vi "LDA_classifier_Trainer_prior.vi"(5 "Matrix":T1, 6 "Non_target_Flash_order":i64[][](array[numeric]) caption="NonTarget_Flash_Order", 7 "Value":T1, 8 "Target_Flash_Order":i64[](array[numeric]), 9 "Brain_data_source":dbl[][](array[numeric]) caption="EEG_Raw_Data" format="%0.3f", 10 "samples per channel":i32=25, 11 "rate":dbl=500.0 caption="Rate" format="%0.2f") -> (0 "FP":dbl[](array[numeric]), 2 "TP":dbl[](array[numeric]))   [LabVIEW 2013]
uses:
  <vilib>/Analysis/Matrix/Datatypes/RealMatrix.ctl
  <vilib>/Analysis/3filter.llb/Filter Passband Type.ctl
  <vilib>/Analysis/baseanly.llb/Mean (DBL).vi
  <vilib>/Analysis/3filter.llb/Butterworth Filter (DBL).vi
  <vilib>/Analysis/Matrix/Numeric/Conversions/Array To Matrix - RA.vi
  <vilib>/Analysis/Matrix/Numeric/Multiply/Multiply - RM,RM.vi
  <vilib>/Analysis/Matrix/Numeric/Subtract/Subtract - RM,RM.vi
  <vilib>/Analysis/Matrix/Numeric/Conversions/Matrix To Array - RM.vi
  <vilib>/Analysis/NI_AALBase.lvlib
  <vilib>/Analysis/Matrix/NI_Matrix.lvlib
panel:
  out "Total Length 2":i32
  out "Total Length":i32
  out "#channel":i32
  out "LDA Parameters\nfor All channel all\nflash":dbl[][](array[numeric])
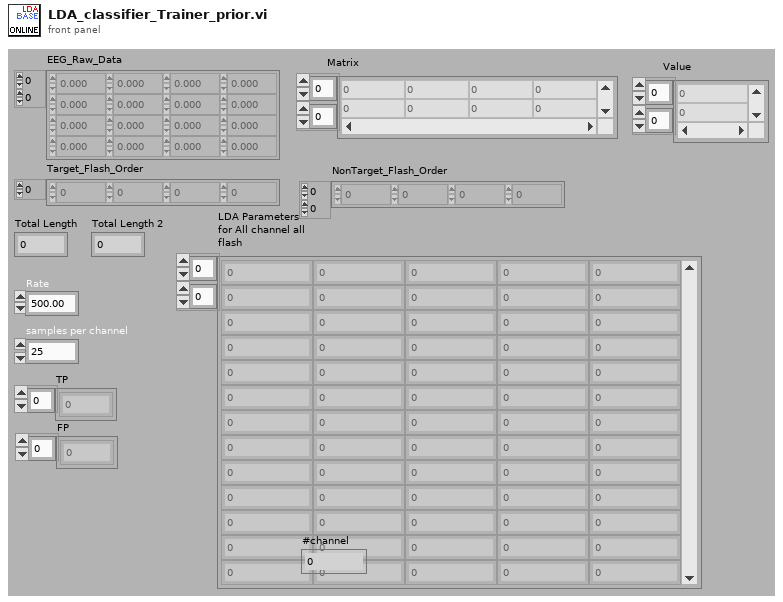
[diagram p1: front panel]
types:
  T1 = typedef "NI_Matrix.lvlib/RealMatrix.ctl" = dbl[][]
  T2 = typedef "NI_AALBase.lvlib/Filter Passband Type.ctl" = enum32{"Lowpass", "Highpass", "Bandpass", "Bandstop"}
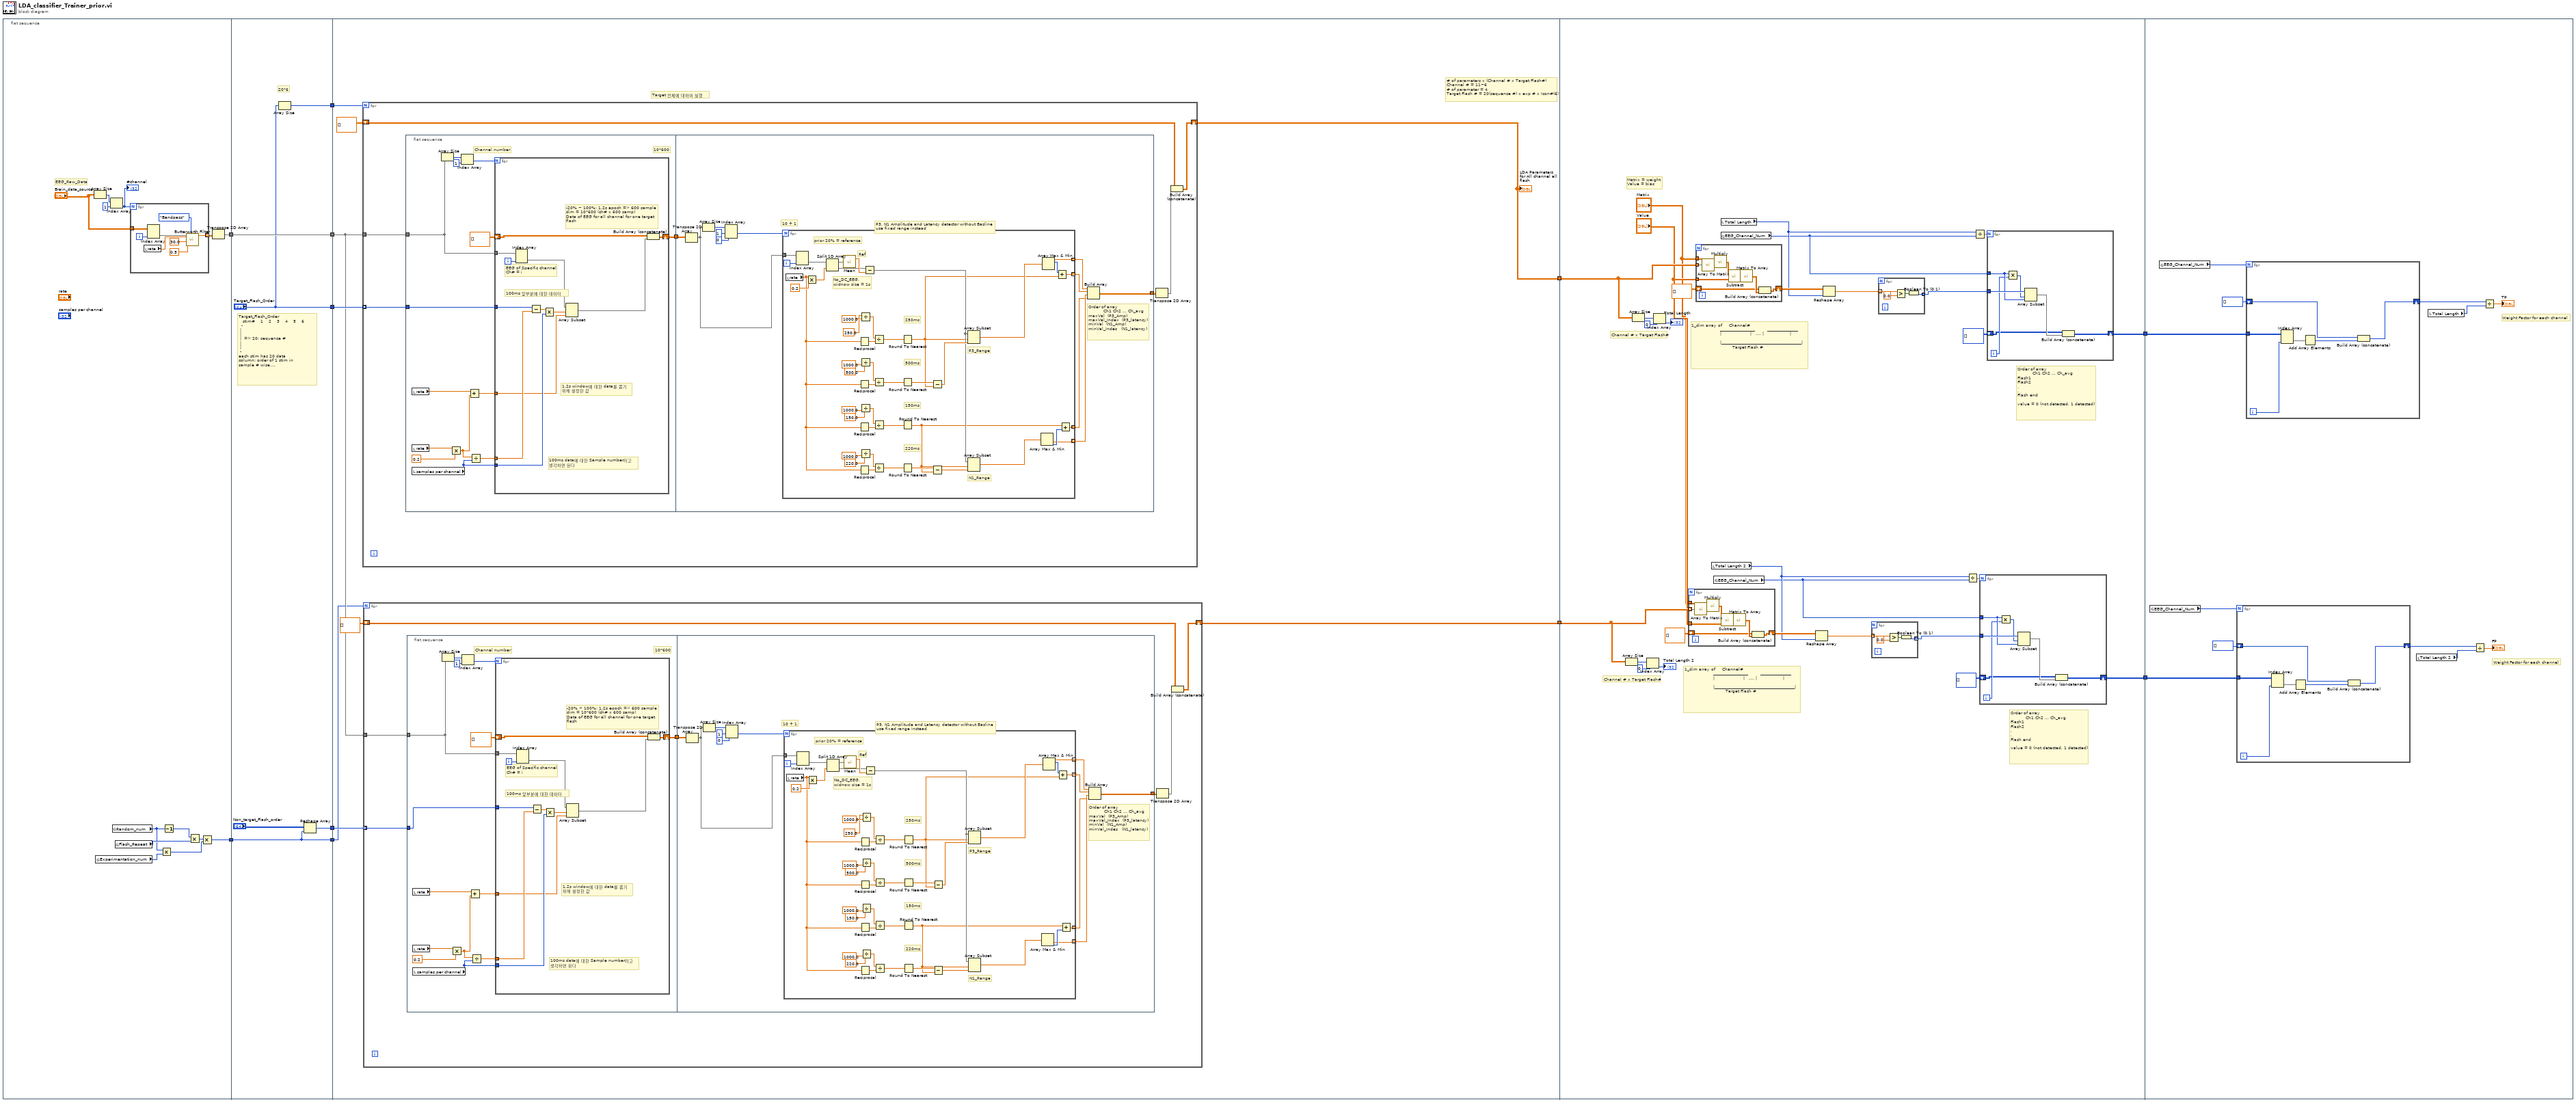
[diagram p0: block diagram]
diagram:
  n1 = flat-sequence {
    tunnel: [w20] -> w11
    tunnel: [w12] -> w2
    tunnel: [w38] -> w10
    tunnel: ["Target_Flash_Order"] -> w9
    tunnel: w11 -> [w38]
    tunnel: [w36] -> w7
    tunnel: [w34] -> w3
    tunnel: w2 -> [w33]
    tunnel: [w33] -> w1
    tunnel: w10 -> [w42]
    tunnel: w9 -> [w47]
    tunnel: [w45] -> w8
    tunnel: w7 -> [w44]
    tunnel: [w41] -> w5
    tunnel: w3 -> [w40]
    tunnel: w1 -> [w39]
    tunnel: w8 -> [w250]
    tunnel: [w239] -> w6
    tunnel: w5 -> [w227]
    tunnel: [w226] -> w4
    tunnel: w6 -> [w303]
    tunnel: w4 -> [w292]
    frame #0 {
      # "EEG_Raw_Data"
      n2 = Array Size(array="Brain_data_source") -> (size(s)=w21:i32[])
      n3 = global read "Control_Panel.vi" "Experimentation_num"() -> (w15:i32)
      n4 = Index Array(array=w21, index=1) -> (element=w23:i32)
      "#channel" <- w23
      n5 = global read "Control_Panel.vi" "Random_num"() -> (w16:i32)
      n6 = global read "Control_Panel.vi" "Flash_Repeat"() -> (w17:i32)
      n7 = for {
        N: w23 -> [_]
        tunnel: "Brain_data_source" -> [w32]
        tunnel: [w28] -> w24 mode=indexing
        i -> [w31]
        n8 = local read "rate"() -> (w25:dbl)
        n9 = Index Array(array=w32, index (col)=w31) -> (element=w30:dbl[])  [unwired: 1 in]
        n10 = call-poly <vilib>:"Butterworth Filter.vi"("filter type"=Filter_Passband_Type."Bandpass", "low cutoff freq: fl"=0.5, "high cutoff freq: fh"=30.0, "sampling freq: fs"=w25, "X"=w30) -> ("Filtered X"=w28:dbl[])  [unwired: 3 in, 1 out]
      }
      n11 = Multiply(x=w16, y=w15) -> (x*y=w13:i32)
      n12 = Decrement(x=w16) -> (x-1=w18:i32)
      n13 = Multiply(x=w18, y=w17) -> (x*y=w14:i32)
      n14 = Multiply(x=w14, y=w13) -> (x*y=w12:i32)
      n15 = Transpose 2D Array(2D array=w24) -> (transposed array=w20:dbl[][])
    }
    frame #1 {
      # "Target_Flash_Order\n   stim#    1    2    3    4    5    6    \n  -\n |\n |\n |  => 20: sequence # \n |\n |\n -\neach stim has 20 data\ncolumn: order of 1 stim in \nsample # wise...."
      # "20*6"
      n16 = Array Size(array="Target_Flash_Order") -> (size(s)=w36:i32)
      n17 = Reshape Array("Non_target_Flash_order", w33) -> (w34:i64[])
    }
    frame #2 {
      # "Target 전체에 대하여 실행"
      # "# of parameters x (Channel # x Target Flash#)\nChannel # = 11~6\n# of parameter = 4\nTarget Flash # = 20(sequence #) x exp # x Icon#(6)"
      n18 = for {
        N: w44 -> [_]
        tunnel: w42 -> [w141]
        tunnel: w47 -> [w136] mode=indexing
        shift-right: [w139] -> w45
        shift-left: dbl[][] [] -> [w138]
        n19 = flat-sequence {
          tunnel: w141 -> [w146]
          tunnel: [w145] -> w142
          tunnel: w136 -> [w144]
          tunnel: w142 -> [w172]
          tunnel: [w174] -> w137
          frame #0 {
            # "10*600"
            # "Channel number"
            n20 = local read "rate"() -> (w154:dbl)
            n21 = local read "rate"() -> (w152:dbl)
            n22 = local read "samples per channel"() -> (w143:i32)
            n23 = Array Size(array=w146) -> (size(s)=w148:i32[])
            n24 = Multiply(x=w152, y=0.2) -> (x*y=w156:dbl)
            n25 = Index Array(array=w148, index=1) -> (element=w150:i32)
            n26 = Add(x=w154, y=w156) -> (x+y=w155:dbl)
            n27 = Divide(x=w156, y=w143) -> (x/y=w153:dbl)
            n28 = for {
              N: w150 -> [_]
              tunnel: w155 -> [w158]
              shift-right: [w166] -> w145
              shift-left: dbl[][] [] -> [w167]
              tunnel: w146 -> [w165]
              tunnel: w153 -> [w162]
              tunnel: w144 -> [w163]
              tunnel: w143 -> [w159]
              i -> [w168]
              # "1.2s window에 대한 data를 뽑기\n위해 설정한 값"
              # "100ms data에 대한 Sample number라고 \n생각하면 된다"
              # "100ms 앞부분에 대한 데이터"
              # "EEG of Specific channel\nCh# = i"
              # "-20% ~ 100%: 1.2s epoch => 600 sample\ndim = 10*600 (ch# x 600 samp)\nData of EEG for all channel for one target \nflash"
              n29 = Index Array(array=w165, index (col)=w168) -> (element=w164:dbl[])  [unwired: 1 in]
              n30 = Subtract(x=w163, y=w162) -> (x-y=w161:dbl)
              n31 = Multiply(x=w161, y=w159) -> (x*y=w160:dbl)
              n32 = Array Subset(array=w164, index=w160, length=w158) -> (w157:dbl[])
              n33 = Build Array (concatenate)(w167, w157) -> (w166:dbl[][])
            }
          }
          frame #1 {
            # "P3, N1 Amplitude and Latency detector without Basline\nuse fixed range instead"
            # "Order of array\n           Ch1 Ch2 ... Ch_avg\nmaxVal  (P3_Amp)\nmaxVal_Index  (P3_latency)\nminVal  (N1_Amp)\nminVal_Indes   (N1_latency)"
            # "10 + 1"
            n34 = Transpose 2D Array(2D array=w172) -> (transposed array=w169:dbl[][])
            n35 = Array Size(array=w169) -> (size(s)=w173:i32[])
            n36 = Index Array(array=w173, index #1=1 ("index"), index #2=0 ("인덱스")) -> (element #1=w170:i32)  [unwired: 1 out]
            n37 = for {
              N: w170 -> [_]
              tunnel: w169 -> [w223]
              tunnel: [w218] -> w178 mode=indexing
              tunnel: [w216] -> w177 mode=indexing
              tunnel: [w213] -> w176 mode=indexing
              tunnel: [w212] -> w175 mode=indexing
              i -> [w211]
              # "N1_Range"
              # "P3_Range"
              # "220ms"
              # "150ms"
              # "500ms"
              # "250ms"
              # "No_DC_EEG,\nwidnow size = 1s"
              # "Ref"
              # "prior 20% = reference"
              n38 = local read "rate"() -> (w193:dbl)
              n39 = Index Array(array=w223, index (col)=w211) -> (element=w215:dbl[])  [unwired: 1 in]
              n40 = Multiply(x=w193, y=0.2) -> (x*y=w221:dbl)
              n41 = Split 1D Array(array=w215, index=w221) -> (first subarray=w220:dbl[], second subarray=w210:dbl[])
              n42 = call-poly <vilib>:"Mean.vi"("X"=w220) -> ("mean"=w219:dbl)  [unwired: 1 out]
              n43 = Reciprocal(x=w193) -> (1/x=w209:dbl)
              n44 = Reciprocal(x=w193) -> (1/x=w208:dbl)
              n45 = Reciprocal(x=w193) -> (1/x=w207:dbl)
              n46 = Reciprocal(x=w193) -> (1/x=w206:dbl)
              n47 = Divide(x=250.0, y=1000.0) -> (x/y=w205:dbl)
              n48 = Divide(x=500.0, y=1000.0) -> (x/y=w204:dbl)
              n49 = Divide(x=150.0, y=1000.0) -> (x/y=w203:dbl)
              n50 = Divide(x=220.0, y=1000.0) -> (x/y=w202:dbl)
              n51 = Subtract(x=w210, y=w219) -> (x-y=w184:dbl[])
              n52 = Divide(x=w205, y=w209) -> (x/y=w192:dbl)
              n53 = Divide(x=w204, y=w208) -> (x/y=w191:dbl)
              n54 = Divide(x=w203, y=w207) -> (x/y=w190:dbl)
              n55 = Divide(x=w202, y=w206) -> (x/y=w189:dbl)
              n56 = Round To Nearest(number=w192) -> (nearest integer value=w181:dbl)
              n57 = Round To Nearest(number=w191) -> (nearest integer value=w186:dbl)
              n58 = Round To Nearest(number=w190) -> (nearest integer value=w180:dbl)
              n59 = Round To Nearest(number=w189) -> (nearest integer value=w188:dbl)
              n60 = Subtract(x=w186, y=w181) -> (x-y=w185:dbl)
              n61 = Subtract(x=w188, y=w180) -> (x-y=w187:dbl)
              n62 = Array Subset(array=w184, index=w181, length=w185) -> (w182:dbl[])
              n63 = Array Subset(array=w184, index=w180, length=w187) -> (w183:dbl[])
              n64 = Array Max & Min(array=w183) -> (min value=w213:dbl, min index (indices)=w214:i32)  [unwired: 2 out]
              n65 = Array Max & Min(array=w182) -> (max value=w218:dbl, max index (indices)=w217:i32)  [unwired: 2 out]
              n66 = Add(x=w217, y=w181) -> (x+y=w216:dbl)
              n67 = Add(x=w180, y=w214) -> (x+y=w212:dbl)
            }
            n68 = Build Array(w178, w177, w176, w175) -> (w174:dbl[][])
          }
        }
        n69 = Transpose 2D Array(2D array=w137) -> (transposed array=w140:dbl[][])
        n70 = Build Array (concatenate)(w138, w140) -> (w139:dbl[][])
      }
      "LDA Parameters\nfor All channel all\nflash" <- w45
      n71 = for {
        N: w39 -> [_]
        tunnel: w42 -> [w53]
        shift-right: [w51] -> w41
        shift-left: dbl[][] [] -> [w50]
        tunnel: w40 -> [w48] mode=indexing
        n72 = flat-sequence {
          tunnel: w53 -> [w58]
          tunnel: [w57] -> w54
          tunnel: w48 -> [w55]
          tunnel: w54 -> [w84]
          tunnel: [w86] -> w49
          frame #0 {
            # "10*600"
            # "Channel number"
            n73 = local read "rate"() -> (w66:dbl)
            n74 = local read "rate"() -> (w64:dbl)
            n75 = local read "samples per channel"() -> (w56:i32)
            n76 = Array Size(array=w58) -> (size(s)=w60:i32[])
            n77 = Multiply(x=w64, y=0.2) -> (x*y=w68:dbl)
            n78 = Index Array(array=w60, index=1) -> (element=w62:i32)
            n79 = Add(x=w66, y=w68) -> (x+y=w67:dbl)
            n80 = Divide(x=w68, y=w56) -> (x/y=w65:dbl)
            n81 = for {
              N: w62 -> [_]
              tunnel: w67 -> [w71]
              shift-right: [w78] -> w57
              shift-left: dbl[][] [] -> [w79]
              tunnel: w58 -> [w77]
              tunnel: w65 -> [w75]
              tunnel: w56 -> [w72]
              tunnel: w55 -> [w69]
              i -> [w80]
              # "1.2s window에 대한 data를 뽑기\n위해 설정한 값"
              # "100ms data에 대한 Sample number라고 \n생각하면 된다"
              # "100ms 앞부분에 대한 데이터"
              # "EEG of Specific channel\nCh# = i"
              # "-20% ~ 100%: 1.2s epoch => 600 sample\ndim = 10*600 (ch# x 600 samp)\nData of EEG for all channel for one target \nflash"
              n82 = Index Array(array=w77, index (col)=w80) -> (element=w76:dbl[])  [unwired: 1 in]
              n83 = Subtract(x=w69, y=w75) -> (x-y=w74:dbl)
              n84 = Multiply(x=w74, y=w72) -> (x*y=w73:dbl)
              n85 = Array Subset(array=w76, index=w73, length=w71) -> (w70:dbl[])
              n86 = Build Array (concatenate)(w79, w70) -> (w78:dbl[][])
            }
          }
          frame #1 {
            # "P3, N1 Amplitude and Latency detector without Basline\nuse fixed range instead"
            # "Order of array\n           Ch1 Ch2 ... Ch_avg\nmaxVal  (P3_Amp)\nmaxVal_Index  (P3_latency)\nminVal  (N1_Amp)\nminVal_Indes   (N1_latency)"
            # "10 + 1"
            n87 = Transpose 2D Array(2D array=w84) -> (transposed array=w81:dbl[][])
            n88 = Array Size(array=w81) -> (size(s)=w85:i32[])
            n89 = Index Array(array=w85, index #1=1 ("index"), index #2=0 ("인덱스")) -> (element #1=w82:i32)  [unwired: 1 out]
            n90 = for {
              N: w82 -> [_]
              tunnel: w81 -> [w135]
              tunnel: [w130] -> w90 mode=indexing
              tunnel: [w128] -> w89 mode=indexing
              tunnel: [w125] -> w88 mode=indexing
              tunnel: [w124] -> w87 mode=indexing
              i -> [w123]
              # "N1_Range"
              # "P3_Range"
              # "220ms"
              # "150ms"
              # "500ms"
              # "250ms"
              # "No_DC_EEG,\nwidnow size = 1s"
              # "Ref"
              # "prior 20% = reference"
              n91 = local read "rate"() -> (w92:dbl)
              n92 = Index Array(array=w135, index (col)=w123) -> (element=w127:dbl[])  [unwired: 1 in]
              n93 = Multiply(x=w92, y=0.2) -> (x*y=w133:dbl)
              n94 = Split 1D Array(array=w127, index=w133) -> (first subarray=w132:dbl[], second subarray=w122:dbl[])
              n95 = call-poly <vilib>:"Mean.vi"("X"=w132) -> ("mean"=w131:dbl)  [unwired: 1 out]
              n96 = Reciprocal(x=w92) -> (1/x=w121:dbl)
              n97 = Reciprocal(x=w92) -> (1/x=w120:dbl)
              n98 = Reciprocal(x=w92) -> (1/x=w119:dbl)
              n99 = Reciprocal(x=w92) -> (1/x=w118:dbl)
              n100 = Divide(x=250.0, y=1000.0) -> (x/y=w117:dbl)
              n101 = Divide(x=500.0, y=1000.0) -> (x/y=w116:dbl)
              n102 = Divide(x=150.0, y=1000.0) -> (x/y=w115:dbl)
              n103 = Divide(x=220.0, y=1000.0) -> (x/y=w114:dbl)
              n104 = Subtract(x=w122, y=w131) -> (x-y=w97:dbl[])
              n105 = Divide(x=w117, y=w121) -> (x/y=w105:dbl)
              n106 = Divide(x=w116, y=w120) -> (x/y=w104:dbl)
              n107 = Divide(x=w115, y=w119) -> (x/y=w103:dbl)
              n108 = Divide(x=w114, y=w118) -> (x/y=w102:dbl)
              n109 = Round To Nearest(number=w105) -> (nearest integer value=w94:dbl)
              n110 = Round To Nearest(number=w104) -> (nearest integer value=w99:dbl)
              n111 = Round To Nearest(number=w103) -> (nearest integer value=w93:dbl)
              n112 = Round To Nearest(number=w102) -> (nearest integer value=w101:dbl)
              n113 = Subtract(x=w99, y=w94) -> (x-y=w98:dbl)
              n114 = Subtract(x=w101, y=w93) -> (x-y=w100:dbl)
              n115 = Array Subset(array=w97, index=w94, length=w98) -> (w95:dbl[])
              n116 = Array Subset(array=w97, index=w93, length=w100) -> (w96:dbl[])
              n117 = Array Max & Min(array=w96) -> (min value=w125:dbl, min index (indices)=w126:i32)  [unwired: 2 out]
              n118 = Array Max & Min(array=w95) -> (max value=w130:dbl, max index (indices)=w129:i32)  [unwired: 2 out]
              n119 = Add(x=w129, y=w94) -> (x+y=w128:dbl)
              n120 = Add(x=w93, y=w126) -> (x+y=w124:dbl)
            }
            n121 = Build Array(w90, w89, w88, w87) -> (w86:dbl[][])
          }
        }
        n122 = Transpose 2D Array(2D array=w49) -> (transposed array=w52:dbl[][])
        n123 = Build Array (concatenate)(w50, w52) -> (w51:dbl[][])
      }
    }
    frame #3 {
      # "Channel # x Target Flash#"
      # "1_dim array of     Channel#\n                     _________________         _______________\n                     |                     |   .... |                   |\n\n                     |_______________________________________|\n                              Target Flash #"
      # "Order of array\n           Ch1 Ch2 ... Ch_avg\nFlash1\nFlash2\n.\n.\nFlash end\n\nvalue = 0 (not detected, 1 detected)"
      # "Channel # x Target Flash#"
      # "1_dim array of     Channel#\n                     _________________         _______________\n                     |                     |   .... |                   |\n\n                     |_______________________________________|\n                              Target Flash #"
      # "Matrix = weight\nValue = bias"
      # "Order of array\n           Ch1 Ch2 ... Ch_avg\nFlash1\nFlash2\n.\n.\nFlash end\n\nvalue = 0 (not detected, 1 detected)"
      n124 = Array Size(array=w227) -> (size(s)=w237:i32[])
      n125 = Array Size(array=w250) -> (size(s)=w249:i32[])
      n126 = Index Array(array=w237, index=0) -> (element=→"Total Length 2":i32)
      n127 = Index Array(array=w249, index=0) -> (element=→"Total Length":i32)
      n128 = for {
        tunnel: "Matrix" -> [w271]
        tunnel: "Value" -> [w268]
        shift-right: [w265] -> w235
        shift-left: dbl[][] [] -> [w264]
        tunnel: w227 -> [w263] mode=indexing
        n129 = call-poly <vilib>:"Array To Matrix.vi"("Real 1D Array"=w263) -> ("Real Matrix (Column Vector)"=w267:T1)
        n130 = call-poly <vilib>:"Multiply.vi"("Real Matrix B"=w267, "Real Matrix A"=w271) -> ("A * B"=w270:T1)
        n131 = call-poly <vilib>:"Subtract.vi"("Real Matrix B"=w268, "Real Matrix A"=w270) -> ("A - B"=w269:T1)
        n132 = call-poly <vilib>:"Matrix To Array.vi"("Real Matrix"=w269) -> ("Real 2D Array"=w266:dbl[][])
        n133 = Build Array (concatenate)(w264, w266) -> (w265:dbl[][])
      }
      n134 = for {
        tunnel: "Matrix" -> [w291]
        tunnel: "Value" -> [w288]
        shift-right: [w285] -> w247
        shift-left: dbl[][] [] -> [w284]
        tunnel: w250 -> [w283] mode=indexing
        n135 = call-poly <vilib>:"Array To Matrix.vi"("Real 1D Array"=w283) -> ("Real Matrix (Column Vector)"=w287:T1)
        n136 = call-poly <vilib>:"Multiply.vi"("Real Matrix B"=w287, "Real Matrix A"=w291) -> ("A * B"=w290:T1)
        n137 = call-poly <vilib>:"Subtract.vi"("Real Matrix B"=w288, "Real Matrix A"=w290) -> ("A - B"=w289:T1)
        n138 = call-poly <vilib>:"Matrix To Array.vi"("Real Matrix"=w289) -> ("Real 2D Array"=w286:dbl[][])
        n139 = Build Array (concatenate)(w284, w286) -> (w285:dbl[][])
      }
      n140 = local read "Total Length 2"() -> (w232:i32)
      n141 = global read "Control_Panel.vi" "EEG_Channel_Num"() -> (w231:i32)
      n142 = local read "Total Length"() -> (w244:i32)
      n143 = global read "Control_Panel.vi" "EEG_Channel_Num"() -> (w243:i32)
      n144 = Reshape Array(w235, w232) -> (w230:dbl[])
      n145 = Reshape Array(w247, w244) -> (w242:dbl[])
      n146 = for {
        tunnel: w230 -> [w255] mode=indexing
        tunnel: [w254] -> w229 mode=indexing
        n147 = Greater?(x=w255, y=0.0) -> (0:w252:bool)
        n148 = Boolean To (0,1)(Boolean=w252) -> (0, 1=w254:i16)
      }
      n149 = for {
        tunnel: w242 -> [w275] mode=indexing
        tunnel: [w274] -> w241 mode=indexing
        n150 = Greater?(x=w275, y=0.0) -> (0:w272:bool)
        n151 = Boolean To (0,1)(Boolean=w272) -> (0, 1=w274:i16)
      }
      n152 = Divide(x=w232, y=w231) -> (x/y=w233:dbl)
      n153 = Divide(x=w244, y=w243) -> (x/y=w245:dbl)
      n154 = for {
        N: w233 -> [_]
        tunnel: w229 -> [w262]
        tunnel: w231 -> [w261]
        shift-right: [w257] -> w226
        shift-left: i16[][] [] -> [w256]
        i -> [w260]
        n155 = Multiply(x=w261, y=w260) -> (x*y=w259:i32)
        n156 = Array Subset(array=w262, index=w259, length=w261) -> (w258:i16[])
        n157 = Build Array (concatenate)(w256, w258) -> (w257:i16[][])
      }
      n158 = for {
        N: w245 -> [_]
        tunnel: w241 -> [w282]
        tunnel: w243 -> [w281]
        shift-right: [w277] -> w239
        shift-left: i16[][] [] -> [w276]
        i -> [w280]
        n159 = Multiply(x=w281, y=w280) -> (x*y=w279:i32)
        n160 = Array Subset(array=w282, index=w279, length=w281) -> (w278:i16[])
        n161 = Build Array (concatenate)(w276, w278) -> (w277:i16[][])
      }
    }
    frame #4 {
      # "Weight Factor for each channel"
      # "Weight Factor for each channel"
      n162 = global read "Control_Panel.vi" "EEG_Channel_Num"() -> (w297:i32)
      n163 = global read "Control_Panel.vi" "EEG_Channel_Num"() -> (w302:i32)
      n164 = for {
        N: w297 -> [_]
        tunnel: w292 -> [w309]
        shift-right: [w305] -> w295
        shift-left: i16[] [] -> [w304]
        i -> [w308]
        n165 = Index Array(array=w309, index (col)=w308) -> (element=w307:i16[])  [unwired: 1 in]
        n166 = Add Array Elements(numeric array=w307) -> (sum=w306:i16)
        n167 = Build Array (concatenate)(w304, w306) -> (w305:i16[])
      }
      n168 = for {
        N: w302 -> [_]
        tunnel: w303 -> [w315]
        shift-right: [w311] -> w300
        shift-left: i16[] [] -> [w310]
        i -> [w314]
        n169 = Index Array(array=w315, index (col)=w314) -> (element=w313:i16[])  [unwired: 1 in]
        n170 = Add Array Elements(numeric array=w313) -> (sum=w312:i16)
        n171 = Build Array (concatenate)(w310, w312) -> (w311:i16[])
      }
      n172 = local read "Total Length 2"() -> (w294:i32)
      n173 = local read "Total Length"() -> (w299:i32)
      n174 = Divide(x=w295, y=w294) -> (x/y=→"FP":dbl[])
      n175 = Divide(x=w300, y=w299) -> (x/y=→"TP":dbl[])
    }
  }
